vi "SetActiveTag__slk_mt.vi"(8 "error in (no error)":errorcluster, 10 "tag":string, 11 "tree view in":refnum<class "TreeView__slk_mt.lvclass">) -> (0 "error out":errorcluster, 2 "duplicated tag":string, 3 "tree view out":refnum<class "TreeView__slk_mt.lvclass">)   [LabVIEW 2020, in "TreeView__slk_mt.lvclass"]
doc: "Sets active tag of a tree view object."
uses:
  TreeView__slk_mt.lvclass
  TreeView__slk_mt.lvclass/TreeView__slk_mt.ctl
panel:
  # "SetActiveTag__slk_mt.vi\nSets active tag of a tree view object.\n\nNOTICE -- YOU MUST LEAVE THIS NOTICE IN PLACE.\n\nCopyright (c) 2011, LIANG LIU Shawn.Liu.cn@gmail.com\nAll rights reserved.\n\nRedistribution and use in source and binary forms, with or without modification, are permitted provided that the following conditions are met:\n-Redistributions of source code must retain the above copyright notice, this list of conditions and the following disclaimer.\n-Redistributions in binary form must reproduce the above copyright notice, this list of conditions and the following disclaimer in the documentation and/or other materials provided with the distribution.\n-Neither the name of the eLp nor the names of its contributors may be used to endorse or promote products derived from this software without specific prior written permission.\n\nTHIS SOFTWARE IS PROVIDED BY THE COPYRIGHT HOLDERS AND CONTRIBUTORS \"AS IS\" AND ANY EXPRESS OR IMPLIED WARRANTIES, INCLUDING, BUT NOT LIMITED TO, THE IMPLIED WARRANTIES OF MERCHANTABILITY AND FITNESS FOR A PARTICULAR PURPOSE ARE DISCLAIMED. IN NO EVENT SHALL THE COPYRIGHT HOLDER OR CONTRIBUTORS BE LIABLE FOR ANY DIRECT, INDIRECT, INCIDENTAL, SPECIAL, EXEMPLARY, OR CONSEQUENTIAL DAMAGES (INCLUDING, BUT NOT LIMITED TO, PROCUREMENT OF SUBSTITUTE GOODS OR SERVICES; LOSS OF USE, DATA, OR PROFITS; OR BUSINESS INTERRUPTION) HOWEVER CAUSED AND ON ANY THEORY OF LIABILITY, WHETHER IN CONTRACT, STRICT LIABILITY, OR TORT (INCLUDING NEGLIGENCE OR OTHERWISE) ARISING IN ANY WAY OUT OF THE USE OF THIS SOFTWARE, EVEN IF ADVISED OF THE POSSIBILITY OF SUCH DAMAGE."
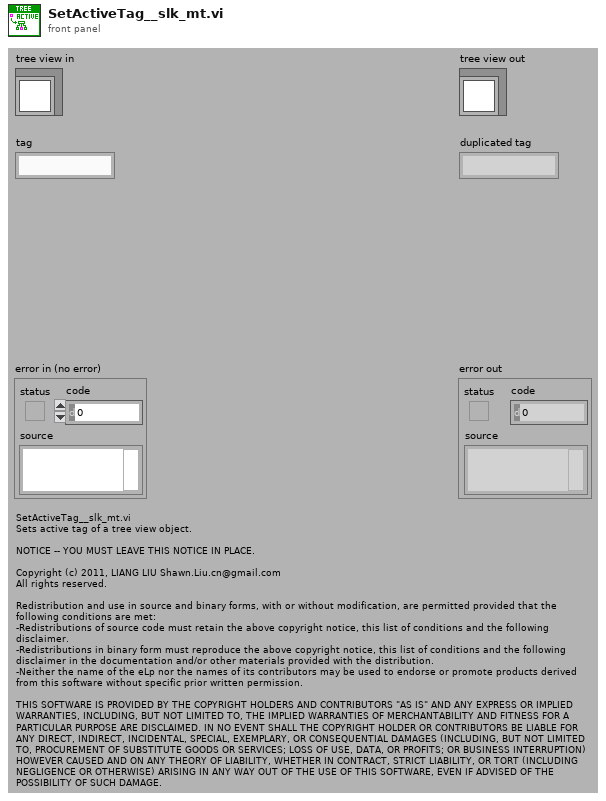
[diagram p1: front panel]
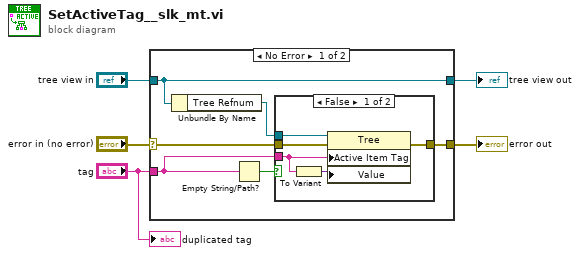
[diagram p0: block diagram]
diagram:
  n1 = case shown="No Error" "error in (no error)" {
    selector: "error in (no error)" -> [w8 w19]
    tunnel: [w9 w19] -> w4
    tunnel: [w11 w18] -> w2
    tunnel: "tree view in" -> [w11 w18]
    tunnel: "tag" -> [w7 _]
    frame No Error {
      n2 = Unbundle By Name(w11) -> ("Tree Refnum"=w10:refnum<vi>)
      n3 = Empty String/Path?(string/path=w7) -> (empty?=w6:bool)
      n4 = case shown="False" w6 {
        tunnel: w10 -> [w16 _]
        tunnel: [w15 w17] -> w9
        tunnel: w8 -> [w14 w17]
        tunnel: w7 -> [w13 _]
        frame False {
          n5 = To Variant(anything=w13) -> (Variant=w12:variant)
          n6 = property class="Tree"(reference=w16, error in=w14, "Active Item Tag"=w13, "Value"=w12) -> (error out=w15:errorcluster)  [unwired: 1 out]
        }
        frame True {
        }
      }
    }
    frame Error {
    }
  }
  "error out" <- w4
  "tree view out" <- w2
  "duplicated tag" <- "tag"
